vi "Set Modules--template.vi"(6 "wait for reply (T)":bool=TRUE, 8 "error in (no error)":errorcluster, 10 "Module Paths":path[](array[path])) -> (0 "error out":errorcluster, 1 "timed out?":bool)   [LabVIEW 2014, in "hse-dqmh-dynamicrequesters.lvlib"]
uses:
  hse-dqmh-dynamicrequesters.lvlib
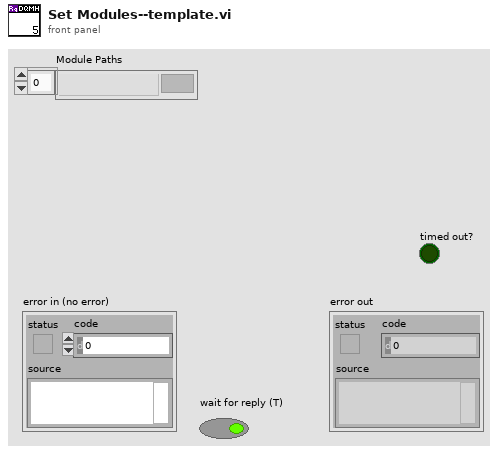
[diagram p1: front panel]
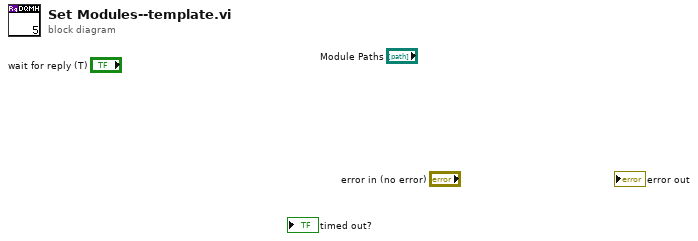
[diagram p0: block diagram]
diagram:
